vi "plot_set_labels.vi"(7 "External PlotObjQueue in":refnum<queue>, 8 "error in (no error)":errorcluster, 9 "label":string, 10 "axis":string(combo)="xlabel", 11 "plot name":string) -> (0 "error out":errorcluster)   [LabVIEW 2017]
doc: "sets the labels of the selected \"axis\" and \"plot\" to \"label\""
uses:
  Classes/Plots/Plots.lvclass
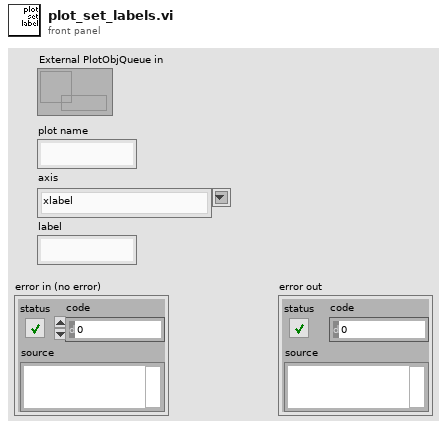
[diagram p1: front panel]
types:
  T1 = cluster{"plot command":string, "Variant":variant}
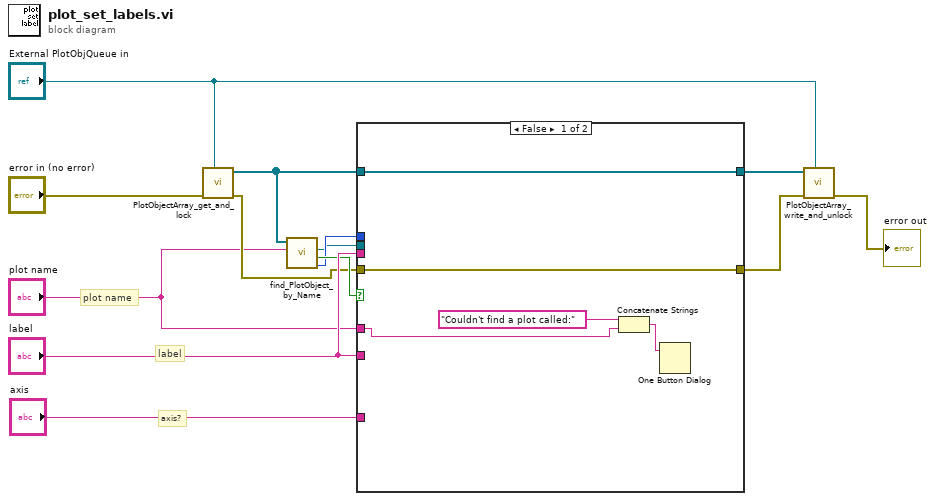
[diagram p0: block diagram]
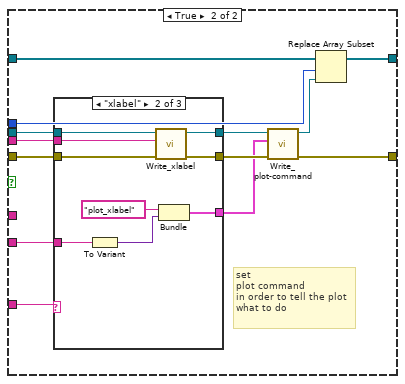
[diagram p2: hidden frame]
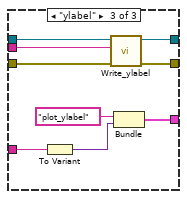
[diagram p4: hidden frame]
diagram:
  # "axis?"
  # "label"
  # "plot name"
  n1 = call "PlotObjectArray_get_and_lock.vi"("External PlotObjQueue in"="External PlotObjQueue in", "error in (no error)"="error in (no error)") -> ("error out"=w9:errorcluster, "PlotObjects"=w6:refnum<class "Plots.lvclass">[])  [unwired: 8 in]
  n2 = call "find_PlotObject_by_Name.vi"("Plot Name/ID"="plot name", "PlotObj Array in"=w6) -> ("index of Object in Array"=w5:i32, "found?"=w12:bool, "found PlotObj out"=w4:refnum<class "Plots.lvclass">)  [unwired: 6 in, 1 out]
  n3 = case shown="False" w12 {
    tunnel: "label" -> [_ w31]
    tunnel: w4 -> [_ w30]
    tunnel: w5 -> [_ w29]
    tunnel: w6 -> [w18 w25]
    tunnel: [w18 w24] -> w7
    tunnel: w9 -> [w17 w23]
    tunnel: [w17 w22] -> w10
    tunnel: "label" -> [_ w21]
    tunnel: "axis" -> [_ w19]
    tunnel: "plot name" -> [w15 _]
    frame False {
      n4 = Concatenate Strings("Couldn't find a plot called:" ("message"), w15) -> (w14:string)
      n5 = One Button Dialog(message=w14) -> ()  [unwired: 1 in, 1 out]
    }
    frame True {
      # "set\nplot command\nin order to tell the plot\nwhat to do"
      n6 = case shown="\"xlabel\"" w19 {
        tunnel: w31 -> [_ w42 w51]
        tunnel: w30 -> [w33 w41 w50]
        tunnel: [w33 w40 w49] -> w28
        tunnel: [w32 w39 w48] -> w26
        tunnel: w23 -> [w32 w38 w47]
        tunnel: w21 -> [_ w36 w45]
        tunnel: [_ w34 w43] -> w20
        frame "", Default {
        }
        frame "xlabel" {
          n7 = To Variant(anything=w36) -> (Variant=w35:variant)
          n8 = call-dynamic "Write_xlabel.vi"("error in (no error)"=w38, "xlabel"=w42, "Plots in"=w41) -> ("error out"=w39:errorcluster, "Plots out"=w40:refnum<class "Plots.lvclass">)  [unwired: 7 in]
          n9 = Bundle("plot command"="plot_xlabel", "Variant"=w35) -> (w34:T1)  [unwired: 1 in]
        }
        frame "ylabel" {
          n10 = To Variant(anything=w45) -> (Variant=w44:variant)
          n11 = call-dynamic "Write_ylabel.vi"("error in (no error)"=w47, "ylabel"=w51, "Plots in"=w50) -> ("error out"=w48:errorcluster, "Plots out"=w49:refnum<class "Plots.lvclass">)  [unwired: 7 in]
          n12 = Bundle("plot command"="plot_ylabel", "Variant"=w44) -> (w43:T1)  [unwired: 1 in]
        }
      }
      n13 = call-dynamic "Write_plot-command.vi"("error in (no error)"=w26, "plot command"=w20, "Plots in"=w28) -> ("error out"=w22:errorcluster, "Plots out"=w27:refnum<class "Plots.lvclass">)  [unwired: 7 in]
      n14 = Replace Array Subset(array=w25, new element=w27, index=w29) -> (w24:refnum<class "Plots.lvclass">[])
    }
  }
  n15 = call "PlotObjectArray_write_and_unlock.vi"("External PlotObjQueue in"="External PlotObjQueue in", "error in (no error)"=w10, "PlotObjects"=w7) -> ("error out"=→"error out":errorcluster)  [unwired: 8 in]
